vi "ui load is jacked.vi"() -> ()   [LabVIEW 2021]
uses:
  <vilib>/Utility/LVLibp/Get Exported File Path.vi
  <vilib>/Utility/LVLibp/Packed Library Path.vi
  src/CIFManagerUI/CIF_Manager_UI.lvclass
  <vilib>/Utility/LVLibp/NI_PackedLibraryUtility.lvlib
panel:
  out "qualified names":string[](array[string])
  out "error out":errorcluster
  in  "packed library path":path=path "C:/Users/Public/Documents/CIF/PluginUI/CIF Template UI.2.0.0.lvlibp"
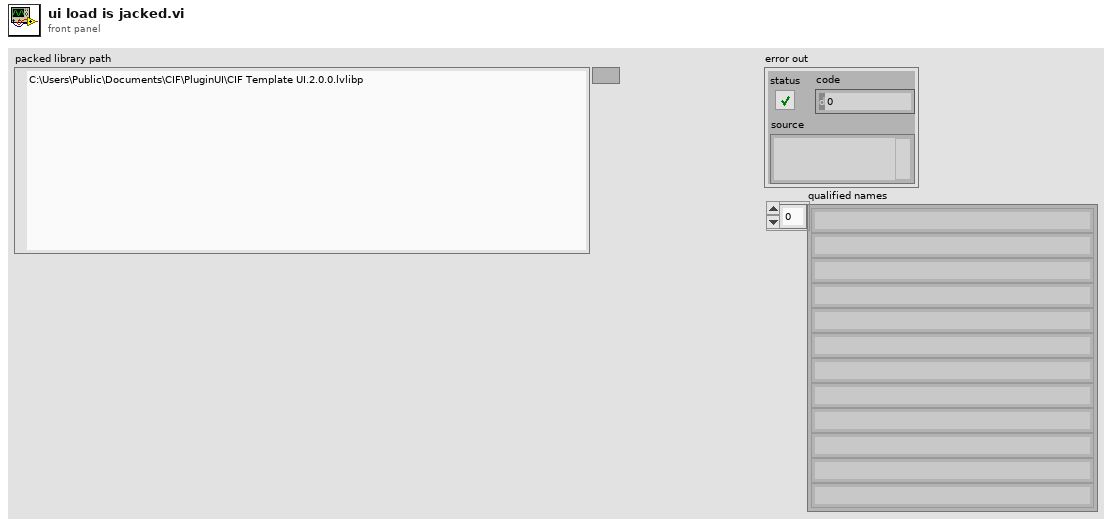
[diagram p1: front panel]
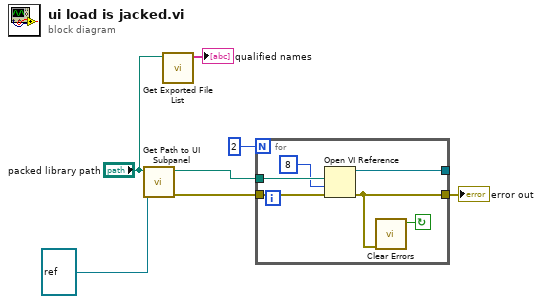
[diagram p0: block diagram]
diagram:
  n1 = call "Get Path to UI Subpanel.vi"("Calling VI"=refnum<vi> refnum, "packed library path"="packed library path") -> ("error out"=w5:errorcluster, "Path to Subpanel"=w6:path)  [unwired: 8 in]
  n2 = call <vilib>:"Get Exported File List.vi"("packed library path"="packed library path") -> ("qualified names"=→"qualified names":string[])  [unwired: 8 in, 2 out]
  n3 = for {
    N: 2 -> [_]
    tunnel: w6 -> [w13]
    tunnel: [w12] -> _
    tunnel: [w11] -> w3
    tunnel: w5 -> [w9]
    stop <- w10 continue-if-true
    n4 = Open VI Reference(vi path=w13, options=8, error in (no error)=w9) -> (vi reference=w12:refnum<vi>, error out=w11:errorcluster)  [unwired: 3 in]
    n5 = call <vilib>:"Clear Errors.vi"("error in (no error)"=w11) -> ("specific error cleared?"=w10:bool)  [unwired: 5 in, 1 out]
  }
  "error out" <- w3
